vi "TimestampsInput.vi"(3 "error in":errorcluster, 4 "FPGA VI Reference In":T1) -> (0 "error out":errorcluster, 1 "Data":u32[](array[numeric]))   [LabVIEW 2011]
uses:
  FPGA_reference.ctl
  <vilib>/Utility/error.llb/Error Cluster From Error Code.vi
  <vilib>/rvi/errors/niLvFpgaAdjustHostInterfaceError.vi
  <vilib>/rvi/interface/nirviMethod/nirviMethod.xnode
  FPGA Bitfiles/FPGA96chmodular3_FPGATarget_fpga8ch-Main_90409DC7.lvbitx
  <vilib>/FPGAPlugInAG/PXI-7813R/niLvFpga_ReadFifo_PXI-7813R.vi
  <vilib>/rvi/errors/niLvFpgaMergeErrorWithErrorCode.vi
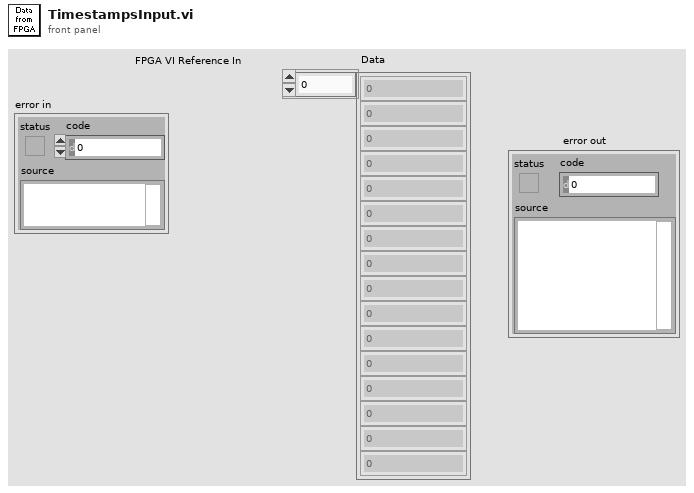
[diagram p1: front panel]
types:
  T1 = typedef "FPGA_reference.ctl" = refnum<k20>
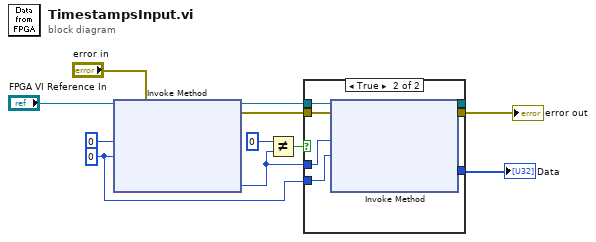
[diagram p0: block diagram]
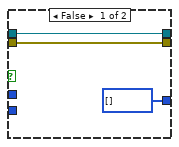
[diagram p2: hidden frame]
diagram:
  w7 = 0 ("Timeout (ms)")
  n1 = xnode "Invoke Method"("FPGA VI Reference In"="FPGA VI Reference In", "error in"="error in", "Number of Elements"=u32 0, "Timeout (ms)"=w7) -> ("FPGA VI Reference Out"=w6:T1, "error out"=w3:errorcluster, "Elements Remaining"=w4:u32)  [unwired: 1 out]
  n2 = Not Equal?(x=u32 0 ("y"), y=w4) -> (x != y?=w11:bool)
  n3 = case shown="True" w11 {
    tunnel: w7 -> [_ w17]
    tunnel: [w12 w21] -> _
    tunnel: [w13 w20] -> w10
    tunnel: w4 -> [_ w19]
    tunnel: w6 -> [w12 w18]
    tunnel: w3 -> [w13 w16]
    tunnel: [u32[] [] ("Data") w15] -> w2
    frame False {
    }
    frame True {
      n4 = xnode "Invoke Method"("FPGA VI Reference In"=w18, "error in"=w16, "Number of Elements"=w19, "Timeout (ms)"=w17) -> ("FPGA VI Reference Out"=w21:T1, "error out"=w20:errorcluster, "Data"=w15:u32[])  [unwired: 1 out]
    }
  }
  "Data" <- w2
  "error out" <- w10
